vi "Ping.vi"(8 "error in (no error)":errorcluster, 11 "test_command":T1) -> (0 "error IO":errorcluster)   [LabVIEW 2018, in "Launcher Main Module.lvlib"]
uses:
  Launcher Main Module.lvlib
  Module_Controls/Test_Command.ctl
  Module_Controls/Test_Response.ctl
  TCP_Write/TCP_Write.lvlib
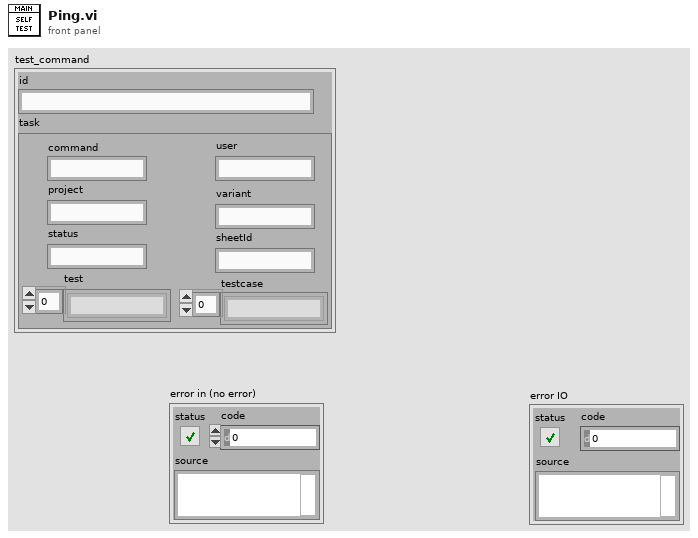
[diagram p1: front panel]
types:
  T1 = typedef "Launcher Main Module.lvlib/Test_Command.ctl" = cluster{"id":string, "task":cluster{"command":string, "project":string, "status":string, "sheetId":string, "test":string[], "user":string, "variant":string, "testcase":string[]}}
  T2 = typedef "Launcher Main Module.lvlib/Test_Response.ctl" = cluster{"id":string, "updates":cluster{"status":string}, "command":string, "project":string, "variant":string, "user":string}
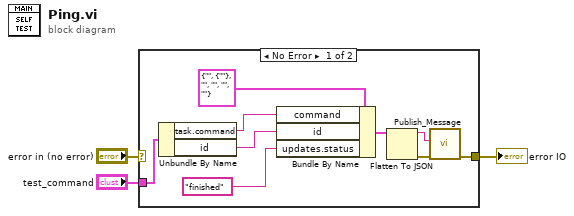
[diagram p0: block diagram]
diagram:
  n1 = case shown="No Error" "error in (no error)" {
    selector: "error in (no error)" -> [_ w13]
    tunnel: [w12 w13] -> w2
    tunnel: "test_command" -> [w10 _]
    frame No Error {
      n2 = Unbundle By Name(w10) -> ("task.command"=w4:string, "id"=w9:string)
      n3 = Bundle By Name(cluster=T2 {"id"="", "updates"={"status"=""}, "command"="", "project"="", "variant"="", "user"=""} ("result"), "command"=w4, "id"=w9, "updates.status"="finished" ("status")) -> (w8:T2)
      n4 = Flatten To JSON(anything=w8) -> (JSON string=w7:string, 11:w6:errorcluster)  [unwired: 2 in]
      n5 = call "Publish_Message.vi"("error in (no error)"=w6, "Publish_Message"=w7) -> ("error out"=w12:errorcluster)  [unwired: 9 in]
    }
    frame Error {
    }
  }
  "error IO" <- w2
